vi "Close Figure.vi"(8 "error in (passthrough)":errorcluster, 11 "reference":refnum<vi>) -> (0 "error out":errorcluster)   [LabVIEW 2020]
uses:
  3e17e1aa-ae8a-4547-ba9d-8b0cd42ca490.vi
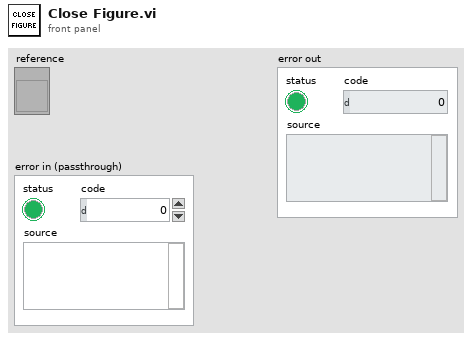
[diagram p1: front panel]
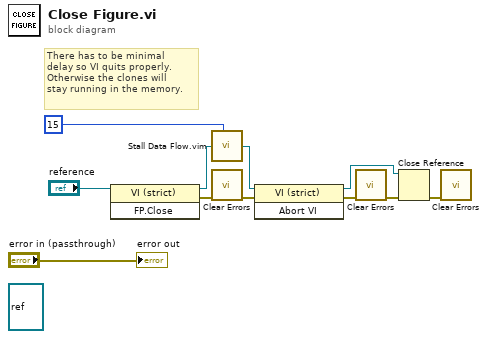
[diagram p0: block diagram]
diagram:
  (unwired) refnum<vi> refnum ("reference out")
  # "There has to be minimal\ndelay so VI quits properly.\nOtherwise the clones will\nstay running in the memory."
  n1 = invoke class="VI (strict)" method="FP.Close"(reference="reference") -> (reference out=w9:refnum<vi>, error out=w5:errorcluster)  [unwired: 2 in, 1 out]
  n2 = call "Stall Data Flow.vim"("value in"=w9, "milliseconds to wait"=u32 15) -> ("value out"=w8:refnum<vi>)  [unwired: 1 out]
  n3 = call <vilib>:"Clear Errors.vi"("error in (no error)"=w5) -> ("error out"=w4:errorcluster)  [unwired: 5 in, 1 out]
  n4 = invoke class="VI (strict)" method="Abort VI"(reference=w8, error in=w4) -> (reference out=w11:refnum<vi>, error out=w3:errorcluster)  [unwired: 1 in, 1 out]
  n5 = call <vilib>:"Clear Errors.vi"("error in (no error)"=w3) -> ("error out"=w2:errorcluster)  [unwired: 5 in, 1 out]
  n6 = Close Reference(reference=w11, error in (no error)=w2) -> (error out=w1:errorcluster)
  n7 = call <vilib>:"Clear Errors.vi"("error in (no error)"=w1) -> ()  [unwired: 5 in, 2 out]
  "error out" <- "error in (passthrough)"
